vi "Read Incoming Bytes.vi"(8 "error in (no error)":errorcluster, 9 "timeout (1000 ms)":i32=1000, 10 "max bytes to read (100000)":i32=100000, 11 "Connection.LocalQueue":refnum<class "Connection.NetworkStream.lvclass">) -> (0 "error out":errorcluster, 1 "timed out":bool, 2 "Bytes":u8[](array[numeric]) format="%08b", 3 "Connection.LocalQueue":refnum<class "Connection.NetworkStream.lvclass">, 4 "connected":bool)   [LabVIEW 2013, in "Connection.NetworkQueue_GOSPL.lvlib" / "Connection.NetworkStream.lvclass"]
uses:
  Connection.NetworkStream/Connection.NetworkStream.lvclass
  Connection.NetworkStream/Connection.NetworkStream.lvclass/Connection.NetworkStream.ctl
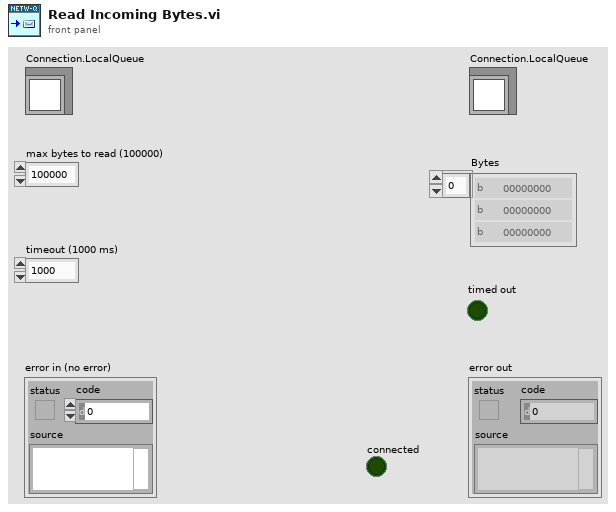
[diagram p1: front panel]
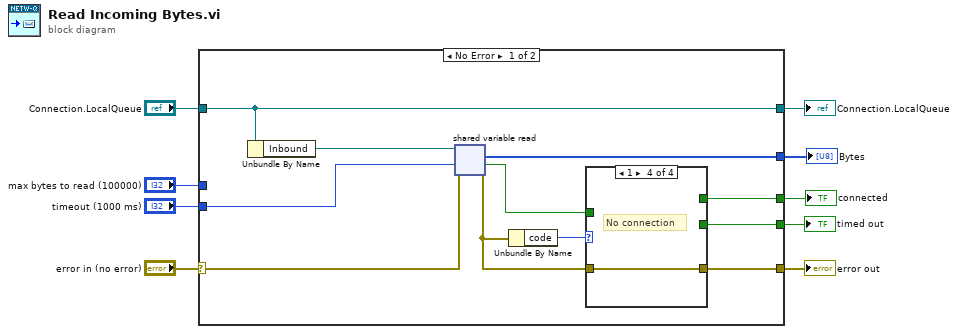
[diagram p0: block diagram]
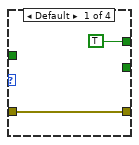
[diagram p2: hidden frame]
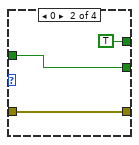
[diagram p3: hidden frame]
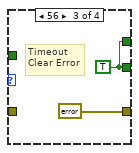
[diagram p4: hidden frame]
diagram:
  n1 = case shown="No Error" "error in (no error)" {
    selector: "error in (no error)" -> [w10 w30]
    tunnel: [w17 w30] -> w8
    tunnel: [w18 w29] -> w6
    tunnel: "Connection.LocalQueue" -> [w18 w29]
    tunnel: [w13 _] -> w5
    tunnel: "max bytes to read (100000)" -> [_ _]
    tunnel: "timeout (1000 ms)" -> [w14 _]
    tunnel: [w19 _] -> w2
    tunnel: [w16 _] -> w1
    frame No Error {
      n2 = Unbundle By Name(w18) -> ("Inbound"=w15:refnum<k21>)
      n3 = shared-variable-read(w15, w10, w14) -> (w11:errorcluster, w12:bool, w13:u8[])  [unwired: 1 out]
      n4 = Unbundle By Name(w11) -> ("code"=w20:i32)
      n5 = case shown="1" w20 {
        tunnel: [w22 w25 errorcluster {"status"=FALSE, "code"=0, "source"=""} ("error out") w28] -> w17
        tunnel: w11 -> [w22 w25 _ w28]
        tunnel: [_ w23 w27 _] -> w19
        tunnel: [TRUE TRUE w27 _] -> w16
        tunnel: w12 -> [_ w23 _ _]
        frame Default {
        }
        frame 0 {
        }
        frame 56 {
          w27 = TRUE
          # "Timeout\nClear Error"
        }
        frame 1 {
          # "No connection"
        }
      }
    }
    frame Error {
    }
  }
  "error out" <- w8
  "Connection.LocalQueue" <- w6
  "Bytes" <- w5
  "timed out" <- w2
  "connected" <- w1
